vi "Write 16bit value.vi"(8 "error in":errorcluster, 9 "value":fxp<+,16,16>, 10 "FPGA Setting":T2, 11 "FPGA ref":T1) -> (0 "error out":errorcluster, 3 "FPGA ref out":T1)   [LabVIEW 2013]
uses:
  FPGA/fpga_settings.ctl
  Scope/controls/settingsFPGAref.ctl
  <vilib>/rvi/interface/common/niFpgaWaitOnOcc.vi
  <vilib>/Utility/error.llb/Error Cluster From Error Code.vi
  <vilib>/rvi/errors/niLvFpgaAdjustHostInterfaceError.vi
  <vilib>/rvi/interface/nirviMethod/nirviMethod.xnode
  <vilib>/FPGAPlugInAG/Dynamic/niLvFpga_WriteFifo_Dynamic.vi
  <vilib>/rvi/errors/niLvFpgaMergeErrorWithErrorCode.vi
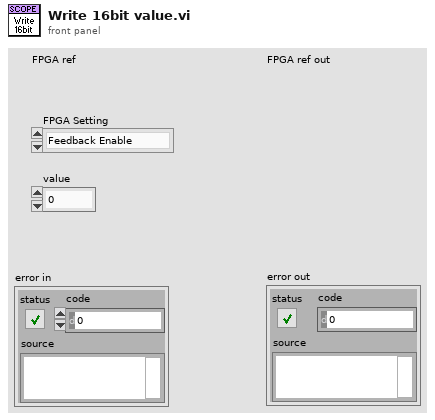
[diagram p1: front panel]
types:
  T1 = typedef "settingsFPGAref.ctl" = refnum<k20>
  T2 = typedef "fpga_settings.ctl" = enum16{"Feedback Enable", "New FIR coeffs", "FIR shift", "Enable filter", "Set Downsample", "Downsample", "CIC Gain", "Record length", "Trigger samples", "Quiet time", "a_am", "b_am", "Use fixed delay", "fixed sin_fi", "fixed cos_fi", "Ki*Tau", "Kp", "Kd_Tau", "Fi_start", "Fi_delta", "DC_offs 0", "DC_offs 1", "Ki*Tau am", "Kp am", "Kd_Tau am"}
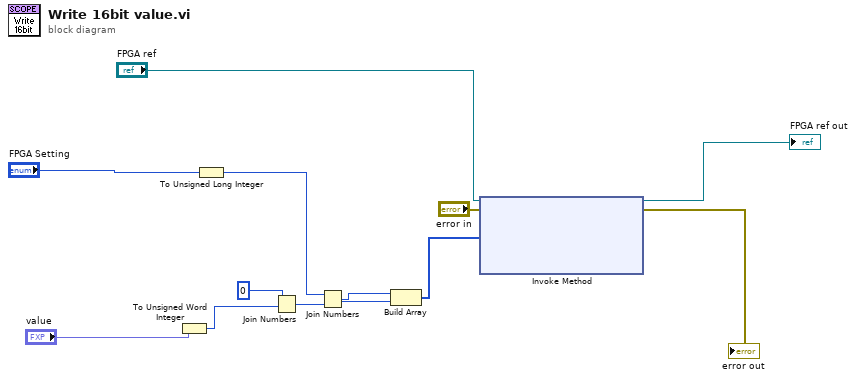
[diagram p0: block diagram]
diagram:
  n1 = To Unsigned Word Integer(number="value") -> (unsigned 16bit integer=w10:u16)
  n2 = To Unsigned Long Integer(number="FPGA Setting") -> (unsigned 32bit integer=w4:u32)
  n3 = Join Numbers(hi=u16 0, lo=w10) -> ((hi.lo)=w11:u32)
  n4 = Join Numbers(hi=w4, lo=w11) -> ((hi.lo)=w3:u64)
  n5 = Build Array(w3, w3) -> (w5:u64[])
  n6 = xnode "Invoke Method"("FPGA VI Reference In"="FPGA ref", "error in"="error in", "Data"=w5) -> ("FPGA VI Reference Out"=→"FPGA ref out":T1, "error out"=→"error out":errorcluster)  [unwired: 1 in, 1 out]
